vi "Move files.vi"(8 "error in (no error)":errorcluster, 9 "source file":path, 10 "Destination directory":path, 11 "Path in":refnum<vi>) -> (0 "error out":errorcluster)   [LabVIEW 2012]
uses:
  <vilib>/Utility/file.llb/Write To Spreadsheet File (string).vi
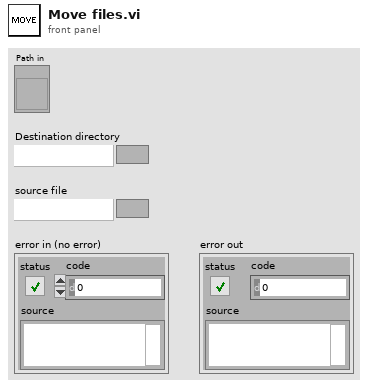
[diagram p1: front panel]
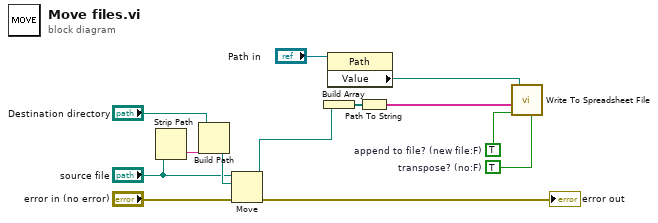
[diagram p0: block diagram]
diagram:
  w7 = TRUE  # transpose? (no:F)
  w8 = TRUE  # append to file? (new file:F)
  n1 = Strip Path(path="source file") -> (name=w5:string)  [unwired: 1 out]
  n2 = Build Path(base path="Destination directory", name or relative path=w5) -> (appended path=w6:path)
  n3 = Move(source path="source file", error in="error in (no error)", 10:w6) -> (error out=→"error out":errorcluster, 3:w9:path)  [unwired: 2 in, 1 out]
  n4 = Build Array(w9) -> (w11:path[])
  n5 = property class="Path"(reference="Path in") -> ("Value"=w12:path)  [unwired: 1 in, 2 out]
  n6 = Path To String(path=w11) -> (string=w10:string[])
  n7 = call-poly <vilib>:"Write To Spreadsheet File.vi"("transpose? (no:F)"=w7, "append to file? (new file:F)"=w8, "1D data"=w10, "file path (dialog if empty)"=w12) -> ()  [unwired: 4 in, 1 out]
